vi "calculate_IQM_MATLAB.vi"(8 "error in (no error)":errorcluster, 9 "Background Value":dbl format="%#_13g", 10 "File Path and Name w/.tif":string="D:\\YD\\test\\FixedCell_groundTruth_crop.tif", 11 "Metrics Type":T1(ring)) -> (0 "error out":errorcluster, 3 "image quality":dbl format="%#_13g")   [LabVIEW 2018]
panel:
  out "mType":i32
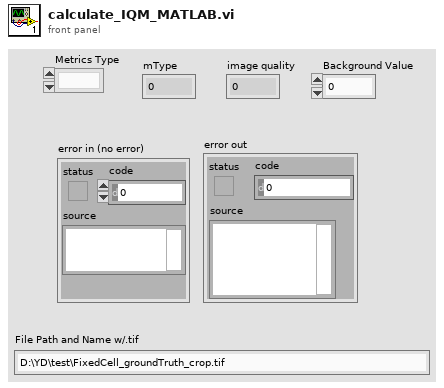
[diagram p1: front panel]
types:
  T1 = enum16{" ", "max intensity", "mean intensity", "RMS contrast", "sharpness - image domain", "sharpness - spectral domain 1: 0~r0", "sharpness - spectral domain 2: 0.1*r0~0.5*r0", "norm DCT  - spectral domain 3: 0~r0"}
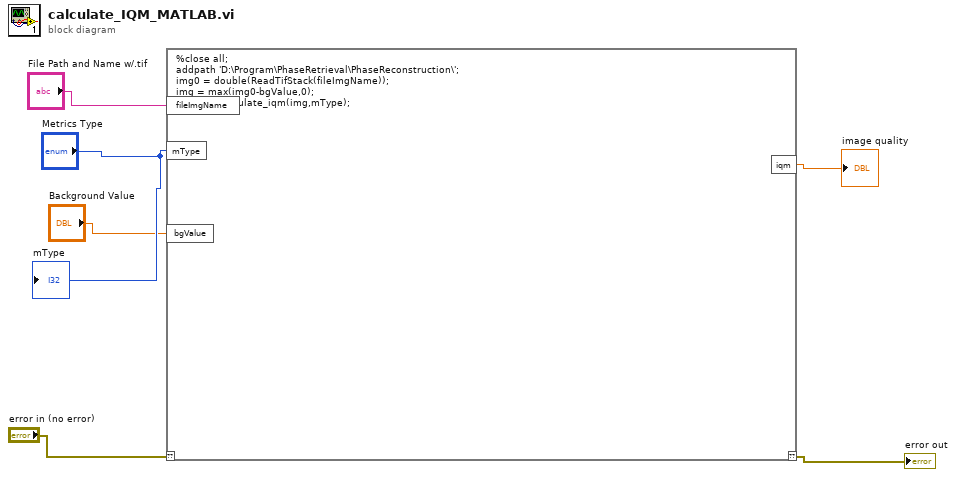
[diagram p0: block diagram]
diagram:
  n1 = script code="%close all;\naddpath 'D:\\Program\\PhaseRetrieval\\PhaseReconstruction\\';\nimg0 = double(ReadTifStack(fileImgName));\nimg = max(img0-bgValue,0);\n[iqm]  = calculate_iqm(img,mType);"("??"="error in (no error)", "fileImgName"="File Path and Name w/.tif", "mType"="Metrics Type", "bgValue"="Background Value") -> ("??"=→"error out":errorcluster, "iqm"=→"image quality":dbl)
  "mType" <- "Metrics Type"
